vi "MM9.set GUI ID.vi"(0 "i ref in":refnum<vi>, 2 "GUIDString":string, 3 "ms timeout (10000)":i32=10000, 5 "error in (no error)":errorcluster) -> (14 "i ref out":refnum<vi>, 17 "timed out":bool, 19 "error out":errorcluster)   [LabVIEW 2014, in "MM9.lvlib"]
doc: "Writes the GUI ID string to the attribute data and publishes it to DIM. A GUI ID string \"N/A\" indicates that no GUI is currently connected."
uses:
  MM9.lvlib
  CSlibraries-extern/DimLVEvent/LVDimInterface/LVDimInterface.lvlib
  CS_Core/CSSystem/CSSystemLib/CSSystemLib.lvlib
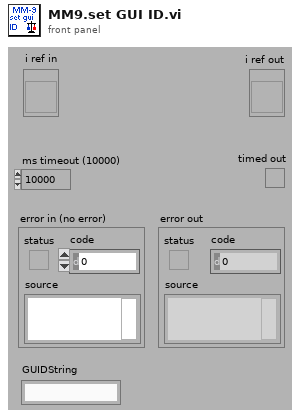
[diagram p1: front panel]
types:
  T1 = typedef "MM9.lvlib/MM9.i attribute.ctl" = cluster{"UsedObjs":string[], "ActScanStep":i32[], "AbortRequest":bool, "StopRequest":bool, "# cycles":i32, "Connected":bool, "MMStatus":T2, "# data":i32, "DIMServices":cluster{"MM6StatusString":string, "MM6StatusID":i32, "discArchiver":string, "discArchiverID":i32, "eventBuilder":string, "eventBuilderID":i32, "GUIIDString":string, "GUIIDStringID":i32}, "dataFile":string, "PGRunning":T3, "ConfigData":T4, "ExtraDataSets":T19}
  T2 = typedef "MM9.lvlib/MM9.status.ctl" = enum16{"loaded", "load_error", "config", "config_error", "init", "init_error", "data_reset", "data_reset_error", "running", "start_error", "run_error", "abort_requested", "aborted", "stop_requested", "stopped", "stop_error", "Connected", "NOTConnected"}
  T3 = typedef "PPG_ABC.lvlib/PPG_ABC.PG_Running.ctl" = i32
  T4 = typedef "LEBITDefs9.lvlib/LEBITDefs.ConfigData.ctl" = cluster{"GenConfig":T5, "Configs":T7[]}
  T5 = typedef "LEBITDefs9.lvlib/LEBITDefs.GenConfig.ctl" = cluster{"Mode":i32, "Logs":T6[]}
  T6 = typedef "LEBITDefs9.lvlib/LEBITDefs.Log.ctl" = cluster{"Name":string, "FctName":string, "Special":string}
  T7 = typedef "LEBITDefs9.lvlib/LEBITDefs.OneConfig.ctl" = cluster{"MCA":T8, "Timing":T9, "Scans":T12[], "FreqDevs":T13[], "CleanDev":T14, "NrCycles":i32, "Specials":T16[], "Delays":T17[], "DAC":T18}
  T8 = typedef "LEBITDefs9.lvlib/LEBITDefs.MCA.ctl" = cluster{"Name":string, "Address":string, "NrChannels":i32, "Gate":i32, "NrPipse":i32, "AcqDelay":i32}
  T9 = typedef "LEBITDefs9.lvlib/LEBITDefs.Timing.ctl" = cluster{"TimeTables":cluster{"TimeTable":T10}[], "Memories":T11[], "ScanX":string, "ScanY":string}
  T10 = typedef "LEBITDefs9.lvlib/LEBITDefs.Timetable.ctl" = dbl[]
  T11 = typedef "LEBITDefs9.lvlib/LEBITDefs.Memory.ctl" = cluster{"Device":string, "ExtTrig":bool, "TT2Use":i32, "PatternTable":string[]}
  T12 = typedef "LEBITDefs9.lvlib/LEBITDefs.ScanDev.ctl" = cluster{"Name":string, "FctName":string, "Values":dbl[], "NrScanVals":i32, "Special":string}
  T13 = typedef "LEBITDefs9.lvlib/LEBITDefs.FreqDev.ctl" = cluster{"Name":string, "Amp":dbl, "CenterFreq":dbl, "Time":dbl}
  T14 = typedef "LEBITDefs9.lvlib/LEBITDefs.CleanDev.ctl" = cluster{"Name":string, "CleanData":T15[]}
  T15 = typedef "LEBITDefs9.lvlib/LEBITDefs.CleanDataType.ctl" = cluster{"Amp":dbl, "Center":dbl, "Plus":dbl, "Minus":dbl, "Time":dbl}
  T16 = typedef "LEBITDefs9.lvlib/LEBITDefs.Special.ctl" = cluster{"Name":string, "FctName":string, "VerySpecial":string, "Data":dbl}
  T17 = typedef "LEBITDefs9.lvlib/LEBITDefs.Delay.ctl" = cluster{"Name":string, "Delay":dbl}
  T18 = typedef "LEBITDefs9.lvlib/LEBITDefs.DAC.ctl" = cluster{"Name":string, "Step1":i32, "Step2":i32}
  T19 = typedef "LEBITDefs9.lvlib/LEBITDefs.ExtraData.ctl" = cluster{"Ions":cluster{"ExcitIonMass":string, "ExcitIonCharge":i32, "CleanIons":cluster{"CleanIonMass":string, "CleanIonCharge":i32}[]}, "TimingDescription":cluster{"TimeTableDescription":cluster{"Times":string[]}[], "PatternTableDescription":cluster{"Pattern":string[]}[]}, "ScanUnits":string[]}[]
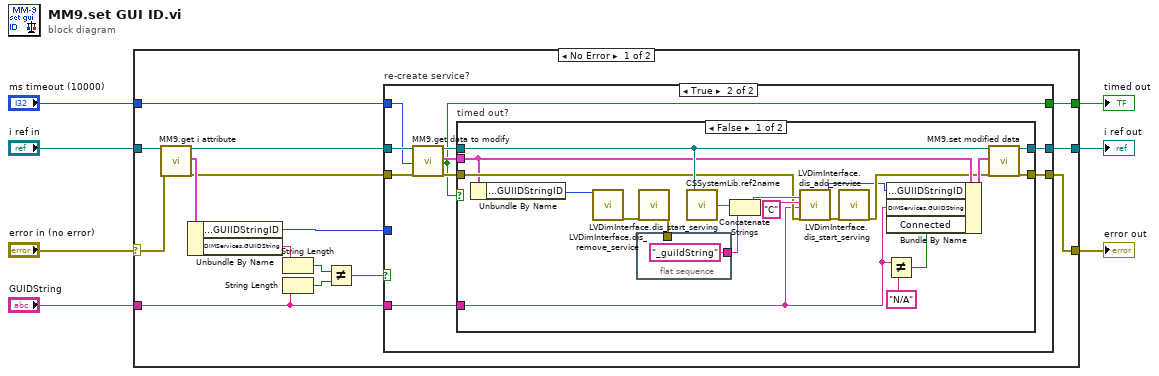
[diagram p0: block diagram]
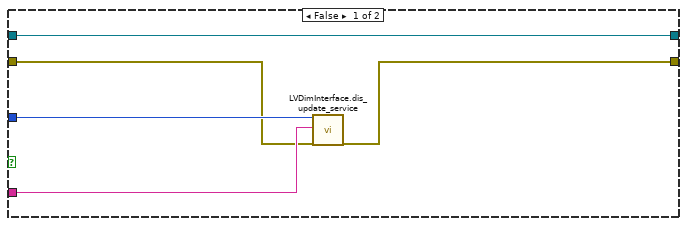
[diagram p2: hidden frame]
diagram:
  n1 = case shown="No Error" "error in (no error)" {
    selector: "error in (no error)" -> [w21 w61]
    tunnel: "i ref in" -> [w22 w60]
    tunnel: [w10 w61] -> w5
    tunnel: [w11 w60] -> w4
    tunnel: "GUIDString" -> [w12 _]
    tunnel: "ms timeout (10000)" -> [w13 _]
    tunnel: [w8 _] -> w1
    frame No Error {
      n2 = call "MM9.get i attribute.vi"("i ref in"=w22, "error in (no error)"=w21) -> ("i ref out"=w15:refnum<vi>, "i attribute"=w20:T1, "error out"=w14:errorcluster)  [unwired: 15 in]
      n3 = Unbundle By Name(w20) -> ("DIMServices.GUIIDStringID"=w9:i32, "DIMServices.GUIIDString"=w18:string)
      n4 = String Length(string=w18) -> (length=w19:i32)
      n5 = String Length(string=w12) -> (length=w17:i32)
      n6 = Not Equal?(x=w19, y=w17) -> (x != y?=w16:bool)
      n7 = case "re-create service?" shown="True" w16 {
        tunnel: w15 -> [w23 w37]
        tunnel: w14 -> [w25 w36]
        tunnel: w13 -> [_ w35]
        tunnel: w12 -> [w26 w32]
        tunnel: [w23 w30] -> w11
        tunnel: [w24 w29] -> w10
        tunnel: w9 -> [w27 _]
        tunnel: [_ w28] -> w8
        frame False {
          n8 = call "LVDimInterface.dis_update_service.vi"("my_serviceID"=w27, "data"=w26, "error in (no error)"=w25) -> ("error out"=w24:errorcluster)  [unwired: 14 in, 2 out]
        }
        frame True {
          n9 = call "MM9.get data to modify.vi"("i ref in"=w37, "ms timeout (10000)"=w35, "error in (no error)"=w36) -> ("i ref out"=w34:refnum<vi>, "i attribute"=w33:T1, "timed out"=w28:bool, "error out"=w31:errorcluster)  [unwired: 13 in]
          n10 = case "timed out?" shown="False" w28 {
            tunnel: w34 -> [w48 w59]
            tunnel: w33 -> [w46 _]
            tunnel: w32 -> [w40 _]
            tunnel: w31 -> [w47 w58]
            tunnel: [w43 w59] -> w30
            tunnel: [w42 w58] -> w29
            frame False {
              n11 = Unbundle By Name(w46) -> ("DIMServices.GUIIDStringID"=w56:i32)
              n12 = call "LVDimInterface.dis_remove_service.vi"("my_serviceID"=w56) -> ("error out"=w55:errorcluster)  [unwired: 18 in]
              n13 = flat-sequence {
                tunnel: ["_guiIdString" ("string")] -> w53
                tunnel: w49 -> [_]
                frame #0 {
                }
              }
              n14 = call "LVDimInterface.dis_start_serving.vi"("error in (no error)"=w55) -> ("error out"=w49:errorcluster)  [unwired: 17 in, 1 out]
              n15 = call "CSSystemLib.ref2name.vi"("obj refnum"=w48) -> ("name"=w54:string)
              n16 = Concatenate Strings(w54, w53) -> (w52:string)
              n17 = call "LVDimInterface.dis_add_service.vi"("serviceName"=w52, "typeDescriptor"="C", "data"=w40, "error in (no error)"=w47) -> ("my_serviceID"=w41:i32, "error out"=w50:errorcluster)  [unwired: 14 in]
              n18 = call "LVDimInterface.dis_start_serving.vi"("error in (no error)"=w50) -> ("error out"=w44:errorcluster)  [unwired: 17 in, 1 out]
              n19 = Not Equal?(x=w40, y="N/A") -> (x != y?=w39:bool)
              n20 = Bundle By Name(cluster=w46, "DIMServices.GUIIDStringID"=w41, "DIMServices.GUIIDString"=w40, "Connected"=w39) -> (w45:T1)
              n21 = call "MM9.set modified data.vi"("i ref in"=w48, "i attribute"=w45, "error in (no error)"=w44) -> ("i ref out"=w43:refnum<vi>, "error out"=w42:errorcluster)  [unwired: 15 in]
            }
            frame True {
            }
          }
        }
      }
    }
    frame Error {
    }
  }
  "error out" <- w5
  "i ref out" <- w4
  "timed out" <- w1
